vi "getGeneralLocation.vi"(8 "error in (no error)":errorcluster, 11 "Idle in":refnum<class "Idle.lvclass">) -> (0 "error out":errorcluster, 2 "General Location":T1 {"North" format="%#_10f"; "East" format="%#_8f"}, 3 "Idle out":refnum<class "Idle.lvclass">)   [LabVIEW 2011, in "Idle.lvclass"]
doc: "Gets the location saved in the class (robot location at mission start) to represent the \"general location\" of this mission."
uses:
  Idle.lvclass
  2 Typedefs/UTM Location.ctl
  Idle.lvclass/Idle.ctl
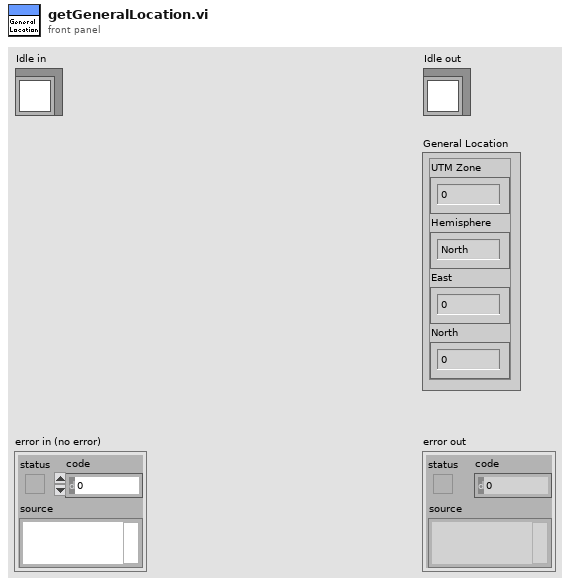
[diagram p1: front panel]
types:
  T1 = typedef "UTM Location.ctl" = cluster{"UTM Zone":dbl, "Hemisphere":enum16{"North", "South"}, "East":dbl, "North":dbl}
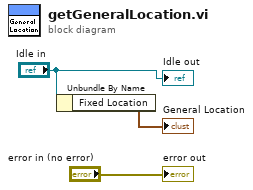
[diagram p0: block diagram]
diagram:
  n1 = Unbundle By Name("Idle in") -> ("Fixed Location"=→"General Location":T1)
  "error out" <- "error in (no error)"
  "Idle out" <- "Idle in"
